vi "计算差值全体均值正图像.vi"(0 "关联成像原理":dbl, 5 "重建方法":dbl, 7 "光源散斑簇":T1, 9 "散斑图像作用结果求和":dbl[](array[numeric]), 11 "散斑图像作用与散斑差分平均值":dbl) -> (4 "未归一化的差值全体均值正图像":dbl[][](array[numeric]))   [LabVIEW 2018]
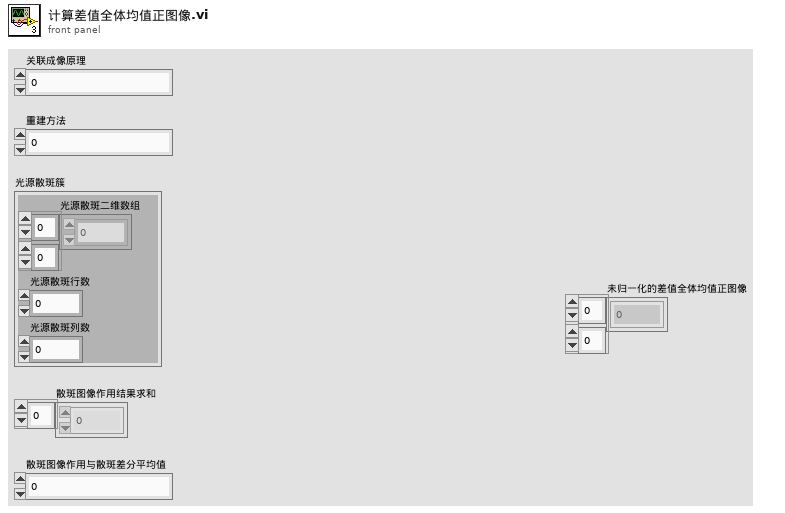
[diagram p1: front panel]
types:
  T1 = cluster{"光源散斑二维数组":dbl[][], "光源散斑行数":i32, "光源散斑列数":i32}
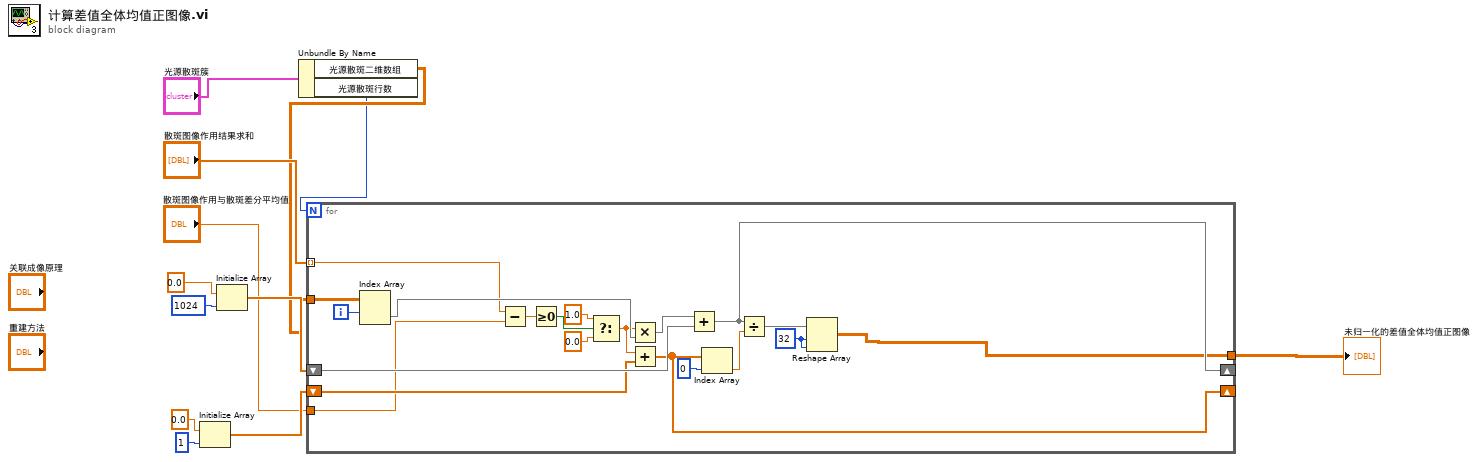
[diagram p0: block diagram]
diagram:
  n1 = Initialize Array(0.0 ("元素"), 1 ("维数大小")) -> (w7:dbl[])
  n2 = Initialize Array(0.0 ("元素"), 1024 ("维数大小")) -> (w8:dbl[])
  n3 = Unbundle By Name("光源散斑簇") -> ("光源散斑二维数组"=w2:dbl[][], "光源散斑行数"=w1:i32)
  n4 = for {
    N: w1 -> [_]
    tunnel: "散斑图像作用与散斑差分平均值" -> [w13]
    tunnel: w2 -> [w32]
    shift-right: [w17] -> _
    shift-left: w8 -> [w24]
    shift-right: [w20] -> _
    shift-left: w7 -> [w23]
    tunnel: [w15] -> w5
    tunnel: "散斑图像作用结果求和" -> [w14] mode=indexing
    i -> [w31]
    w21 = 32 ("维数大小")
    n5 = Index Array(array=w32, index (row)=w31) -> (element=w26:dbl[])  [unwired: 1 in]
    n6 = Subtract(x=w14, y=w13) -> (x-y=w27:dbl)
    n7 = Greater Or Equal To 0?(x=w27) -> (x >= 0?=w30:bool)
    n8 = Select(t=1.0, s=w30, f=0.0) -> (s? t:f=w22:dbl)
    n9 = Multiply(x=w22, y=w26) -> (x*y=w25:dbl[])
    n10 = Add(x=w22, y=w23) -> (x+y=w20:dbl[])
    n11 = Add(x=w25, y=w24) -> (x+y=w17:dbl[])
    n12 = Index Array(array=w20, index=0 ("索引")) -> (element=w18:dbl)
    n13 = Divide(x=w17, y=w18) -> (x/y=w16:dbl[])
    n14 = Reshape Array(w16, w21, w21) -> (w15:dbl[][])
  }
  "未归一化的差值全体均值正图像" <- w5
